vi "Guess Current.vi"(8 "error in (no error)":errorcluster, 9 "Current guess":dbl, 10 "Desired Field":dbl, 11 "Magna Power in":refnum<class "Magna Power.lvclass">) -> (0 "error out":errorcluster, 1 "Stop?":bool, 2 "New guess":dbl, 3 "Magna Power out":refnum<class "Magna Power.lvclass">)   [LabVIEW 2012, in "Magna Power.lvclass"]
doc: "Desired field: assumes a POSITIVE input.\nCurrent guess: the current that has recently been sent to the power supply.\n\nThis VI is for use when the actual field is close (within about 0.02 T) to the desired value. It makes a new guess for the current using derivatives, taking into account the orientation of the leads. It also outputs whether the field has gotten sufficiently close (within 1 mT) to the desired value, indicated by the Stop? output."
uses:
  Magna Power.lvclass
  Magna Power.lvclass/Magna Power.ctl
  Magna Power Constants.vi
  <vilib>/gmath/NI_Gmath.lvlib
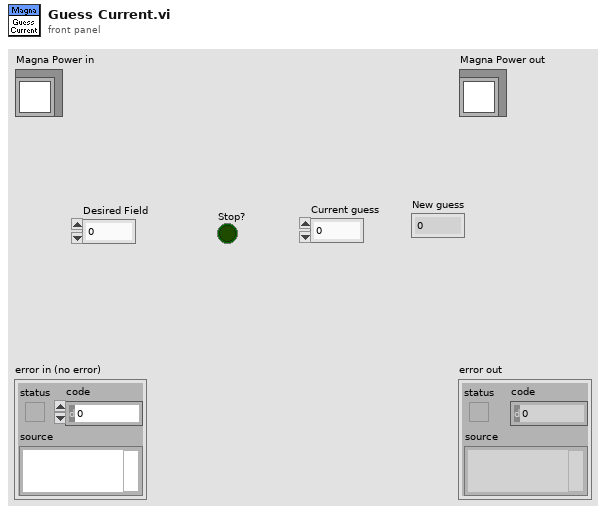
[diagram p1: front panel]
types:
  T1 = cluster{"Field":dbl[], "Current Derivative":dbl[]}
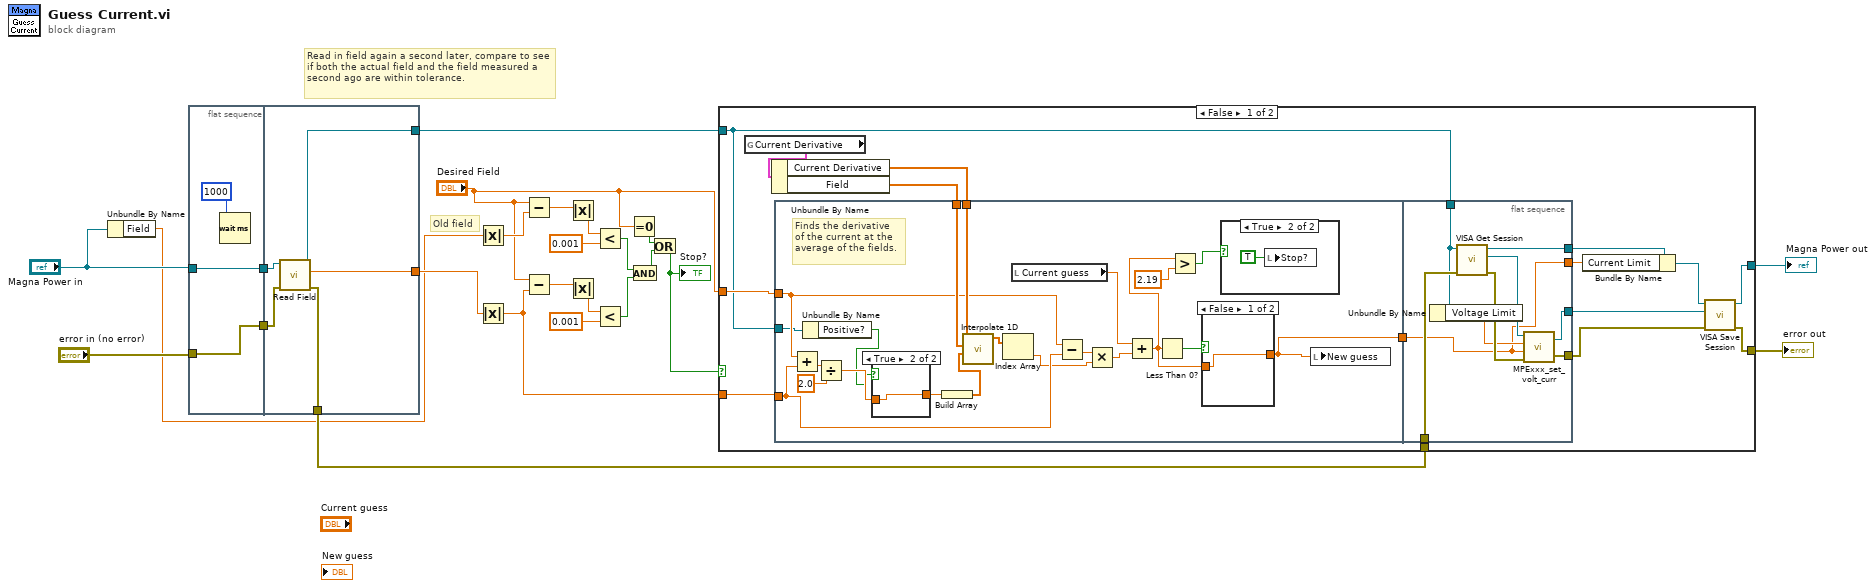
[diagram p0: block diagram]
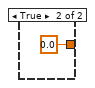
[diagram p3: hidden frame]
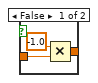
[diagram p4: hidden frame]
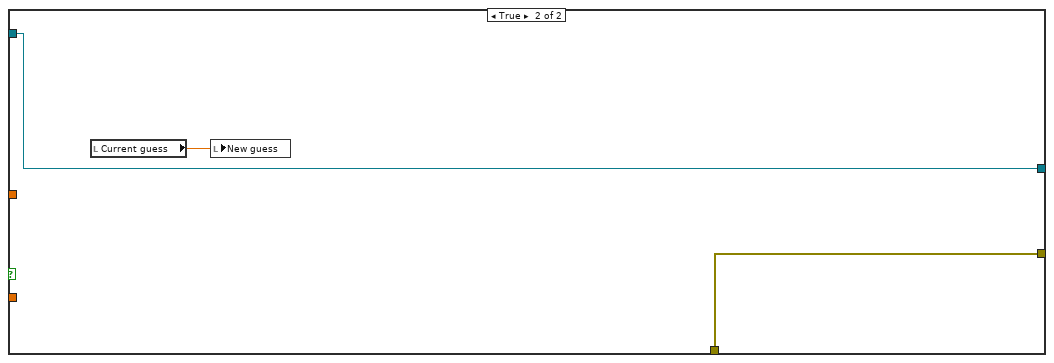
[diagram p5: hidden frame]
diagram:
  # "Old field"
  # "Read in field again a second later, compare to see if both the actual field and the field measured a second ago are within tolerance."
  n1 = Unbundle By Name("Magna Power in") -> ("Field"=w5:dbl)
  n2 = flat-sequence {
    tunnel: [w26] -> w24
    tunnel: "error in (no error)" -> [w26]
    tunnel: [w25] -> w9
    tunnel: "Magna Power in" -> [w25]
    tunnel: w24 -> [w32]
    tunnel: [w31] -> w22
    tunnel: [w30] -> w7
    tunnel: [w29] -> w15
    tunnel: w9 -> [w28]
    frame #0 {
      n3 = Wait (ms)(milliseconds to wait=u32 1000) -> ()  [unwired: 1 out]
    }
    frame #1 {
      n4 = call "Read Field.vi"("error in (no error)"=w32, "Magna Power in"=w28) -> ("error out"=w30:errorcluster, "Field (T)"=w29:dbl, "Magna Power out"=w31:refnum<class "Magna Power.lvclass">)  [unwired: 5 in, 2 out]
    }
  }
  n5 = Absolute Value(x=w5) -> (abs(x)=w21:dbl)
  n6 = Absolute Value(x=w15) -> (abs(x)=w12:dbl)
  n7 = Subtract(x="Desired Field", y=w21) -> (x-y=w20:dbl)
  n8 = Subtract(x="Desired Field", y=w12) -> (x-y=w17:dbl)
  n9 = Absolute Value(x=w20) -> (abs(x)=w19:dbl)
  n10 = Absolute Value(x=w17) -> (abs(x)=w18:dbl)
  n11 = Less?(x=w19, y=0.001) -> (x < y?=w14:bool)
  n12 = Less?(x=w18, y=0.001) -> (x < y?=w13:bool)
  n13 = Equal To 0?(x="Desired Field") -> (x = 0?=w2:bool)
  n14 = And(x=w14, y=w13) -> (x .and. y?=w3:bool)
  n15 = Or(x=w2, y=w3) -> (x .or. y?=w1:bool)
  "Stop?" <- w1
  n16 = case shown="False" w1 {
    tunnel: [w35 w85] -> w10
    tunnel: w12 -> [w43 _]
    tunnel: "Desired Field" -> [w42 _]
    tunnel: w22 -> [w38 w86]
    tunnel: [w36 w86] -> w8
    tunnel: w7 -> [w41 w85]
    frame False {
      n17 = global read "Magna Power Constants.vi" "Current Derivative"() -> (w44:T1)
      n18 = Unbundle By Name(w44) -> ("Current Derivative"=w45:dbl[], "Field"=w46:dbl[])
      n19 = flat-sequence {
        tunnel: w46 -> [w66]
        tunnel: w45 -> [w65]
        tunnel: w43 -> [w59]
        tunnel: w42 -> [w60]
        tunnel: [w54] -> w47
        tunnel: w38 -> [w49]
        tunnel: w47 -> [w76]
        tunnel: [w84] -> w40
        tunnel: w38 -> [w78]
        tunnel: w41 -> [w83]
        tunnel: [w80] -> w39
        tunnel: [w79] -> w34
        tunnel: [w76] -> w33
        frame #0 {
          # "Finds the derivative\nof the current at the\naverage of the fields."
          n20 = Add(x=w60, y=w59) -> (x+y=w63:dbl)
          n21 = Unbundle By Name(w49) -> ("Positive?"=w48:bool)
          n22 = Divide(x=w63, y=2.0) -> (x/y=w61:dbl)
          n23 = case shown="True" w48 {
            tunnel: w61 -> [w73 w75]
            tunnel: [w72 w75] -> w68
            frame False {
              n24 = Multiply(x=-1.0, y=w73) -> (x*y=w72:dbl)
            }
            frame True {
            }
          }
          n25 = Build Array(w68) -> (w67:dbl[])
          n26 = call <vilib>:"Interpolate 1D.vi"("xi"=w67, "X"=w66, "Y"=w65) -> ("yi"=w64:dbl[])  [unwired: 6 in, 2 out]
          n27 = Index Array(array=w64) -> (element=w57:dbl)  [unwired: 1 in]
          n28 = local read "Current guess"() -> (w52:dbl)
          n29 = Subtract(x=w60, y=w59) -> (x-y=w58:dbl)
          n30 = Multiply(x=w58, y=w57) -> (x*y=w56:dbl)
          n31 = Add(x=w52, y=w56) -> (x+y=w50:dbl)
          n32 = Less Than 0?(x=w50) -> (x < 0?=w55:bool)
          n33 = Greater?(x=w50, y=2.19 ("x")) -> (0:w53:bool)
          n34 = case shown="False" w55 {
            tunnel: [w70 0.0] -> w54
            tunnel: w50 -> [w70 _]
            frame False {
            }
            frame True {
            }
          }
          n35 = case shown="True" w53 {
            frame False {
            }
            frame True {
              n36 = local write "Stop?"(TRUE ("Stop?")) -> ()
            }
          }
          n37 = local write "New guess"(w54) -> ()
        }
        frame #1 {
          n38 = Unbundle By Name(w78) -> ("Voltage Limit"=w77:dbl)
          n39 = call-dynamic "VISA Get Session.vi"("error in (no error)"=w83, "Instrument.lvclass in"=w78) -> ("error out"=w82:errorcluster, "VISA Resource Name"=w81:refnum<visa-resource-name>, "Instrument.lvclass out"=w79:refnum<class "Magna Power.lvclass">)  [unwired: 6 in, 1 out]
          n40 = call "MPExxx_set_volt_curr.vi"("error in (no error)"=w82, "Set Current"=w76, "Set Voltage"=w77, "VISA session"=w81) -> ("error out"=w84:errorcluster, "dup VISA session"=w80:refnum<visa-resource-name>)
        }
      }
      n41 = Bundle By Name(cluster=w34, "Current Limit"=w33) -> (w37:refnum<class "Magna Power.lvclass">)
      n42 = call-dynamic "VISA Save Session.vi"("error in (no error)"=w40, "VISA Resource Name"=w39, "Instrument.lvclass in"=w37) -> ("error out"=w35:errorcluster, "Instrument.lvclass out"=w36:refnum<class "Magna Power.lvclass">)  [unwired: 7 in]
    }
    frame True {
      n43 = local read "Current guess"() -> (w87:dbl)
      n44 = local write "New guess"(w87) -> ()
    }
  }
  "error out" <- w10
  "Magna Power out" <- w8
